vi "TPNPT_MinorFilter.vi"(0 "Values":dbl[](array[numeric]) format="%.2f", 1 "last value":dbl format="%.2f", 2 "Number of samples":i32, 4 "index":i32) -> (7 "average":dbl format="%.2f", 8 "Values out":dbl[](array[numeric]) format="%.2f")   [LabVIEW 2016]
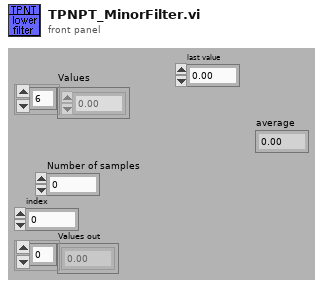
[diagram p1: front panel]
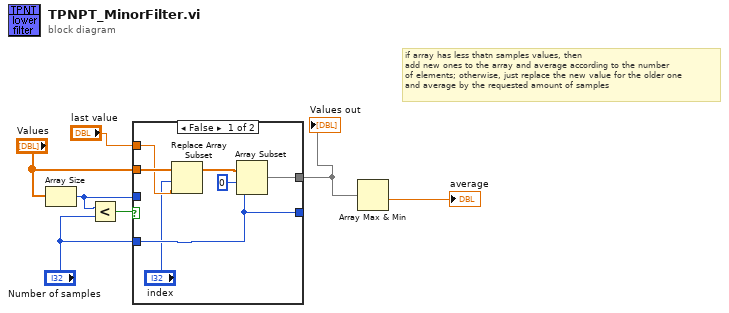
[diagram p0: block diagram]
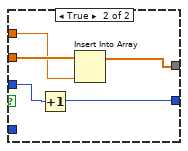
[diagram p2: hidden frame]
diagram:
  # "if array has less thatn samples values, then\nadd new ones to the array and average according to the number\nof elements; otherwise, just replace the new value for the older one\nand average by the requested amount of samples"
  n1 = Array Size(array="Values") -> (size(s)=w3:i32)
  n2 = Less?(x=w3, y="Number of samples") -> (x < y?=w5:bool)
  n3 = case shown="False" w5 {
    tunnel: [w13 w17] -> w2
    tunnel: "Values" -> [w11 w19]
    tunnel: [w12 w15] -> _
    tunnel: "Number of samples" -> [w12 _]
    tunnel: "last value" -> [w9 w18]
    tunnel: w3 -> [_ w16]
    frame False {
      n4 = Replace Array Subset(array=w11, new element=w9, index="index") -> (w10:dbl[])
      n5 = Array Subset(array=w10, index=0 ("Array Index"), length=w12) -> (w13:dbl[])
    }
    frame True {
      n6 = Increment(x=w16) -> (x+1=w15:i32)
      n7 = Insert Into Array(array=w19, new element=w18) -> (w17:dbl[])  [unwired: 1 in]
    }
  }
  "Values out" <- w2
  n8 = Array Max & Min(array=w2) -> (min value=→"average":dbl)  [unwired: 3 out]
